vi "Configure Acquisition.vi"(8 "error in":errorcluster, 11 "Scope PXI CFG in":refnum<class "Scope PXI CFG.lvclass">) -> (0 "error out":errorcluster, 3 "Scope PXI CFG out":refnum<class "Scope PXI CFG.lvclass">)   [LabVIEW 2023, in "Scope.lvlib" / "Scope PXI.lvlib" / "Scope PXI CFG.lvclass"]
uses:
  Scope PXI CFG.lvclass
  <instrlib>/niScope/Controls/niScope acquisition type.ctl
  Scope PXI CFG.lvclass/Scope PXI CFG.ctl
  Configuration Base/Configuration Base.lvclass/Configuration Base.ctl
  33e6a676-ff2b-4197-9c74-0448942d65be.vi
  <vilib>/JDP Science/JSONtext/Next JSON Value.vi
  <vilib>/JDP Science/JSONtext/String Subset.vi
  <vilib>/JDP Science/JSONtext/Parsing/Advance past next JSON Value (inlined COPY).vi
  <vilib>/JDP Science/JSONtext/Parsing/Advance past whitespace.vi
  <vilib>/JDP Science/JSONtext/Parsing/Advance past String.vi
  <vilib>/JDP Science/JSONtext/Parsing/Advance past Number.vi
  <vilib>/JDP Science/JSONtext/Parsing/Advance past Line Ending.vi
  <vilib>/JDP Science/JSONtext/Parsing/Parse Full Path or Item Name.vi
  <vilib>/JDP Science/JSONtext/Parsing/Advance past Array.vi
  <vilib>/JDP Science/JSONtext/Parsing/Advance past Object.vi
  <vilib>/JDP Science/JSONtext/support/Error Cluster From Code.vi
  <vilib>/JDP Science/JSONtext/Offset/Find Item Locations by Path.vi
  <vilib>/JDP Science/JSONtext/JSON text to Variant.vi
  <vilib>/Utility/error.llb/Error Cluster From Error Code.vi
  <vilib>/JDP Science/JSONtext/LVClass Serializer/JSONtext LVClass Serializer.lvclass
  <vilib>/ErrorRing/Error Ring.xnode
  Configuration Base/Configuration Base.lvclass
  <vilib>/JDP Science/JSONtext/JSONtext.lvlib
panel:
  out "acquisition Type":T1 caption="acquisition type (Normal)" items=["Normal"=0, "Flex Res"=1, "DDC"=3]
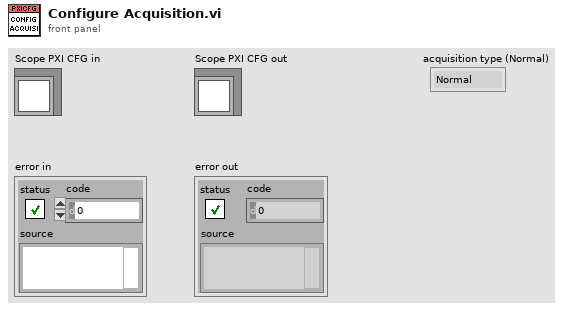
[diagram p1: front panel]
types:
  T1 = typedef "niScope acquisition type.ctl" = i32
  T2 = typedef "LVStringsAndValuesArrayTypeDef_I32.ctl" = cluster{"String":string, "Value":i32}[]
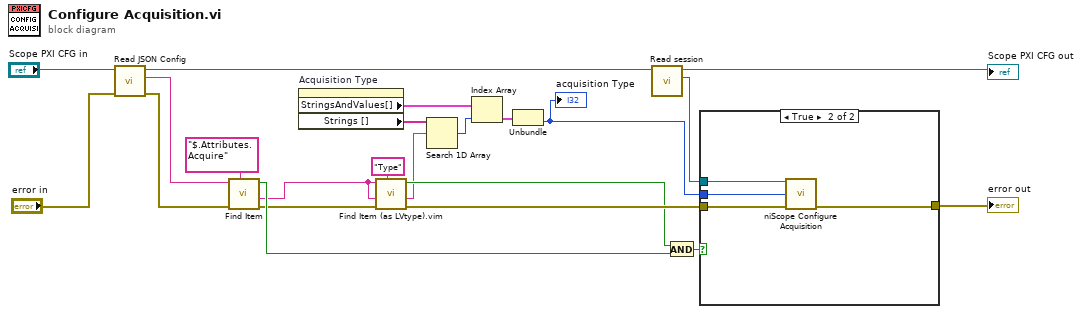
[diagram p0: block diagram]
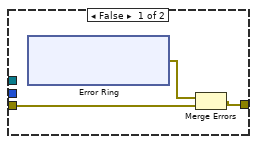
[diagram p2: hidden frame]
diagram:
  n1 = call "Read JSON Config.vi"("error in"="error in", "object in"="Scope PXI CFG in") -> ("error out"=w20:errorcluster, "<JSON>Config"=w21:string, "object out"=w22:refnum<class "Scope PXI CFG.lvclass">)  [unwired: 7 in]
  n2 = call <vilib>:"Find Item.vi"("$Path or Item Name"="$.Attributes.Acquire", "error in (no error)"=w20, "JSON"=w21) -> ("error out"=w17:errorcluster, "<JSON>"=w1:string, "Found"=w19:bool)  [unwired: 5 in, 1 out]
  n3 = property on="Acquisition Type" class="Ring (strict)"() -> ("StringsAndValues[]"=w5:T2, "Strings []"=w7:string[])  [unwired: 2 in, 2 out]
  n4 = call "Find Item (as LVtype).vim"("$Path or Item Name"="Type", "error in (no error)"=w17, "Data Type and Default Value"=w1, "JSON"=w1) -> ("error out"=w14:errorcluster, "Data"=w6:string, "Found"=w13:bool)  [unwired: 4 in, 1 out]
  n5 = Search 1D Array(1D array=w7, element=w6) -> (index of element=w4:i32)  [unwired: 1 in]
  n6 = Index Array(array=w5, index=w4) -> (element=w3:cluster{"String":string, "Value":i32})
  n7 = Unbundle(w3) -> ("Value"=w2:i32)  [unwired: 1 out]
  "acquisition Type" <- w2
  n8 = call "Read session.vi"("Scope PXI CFG in"=w22) -> ("session"=w16:refnum<k15>, "Scope PXI CFG out"=→"Scope PXI CFG out":refnum<class "Scope PXI CFG.lvclass">)  [unwired: 8 in, 1 out]
  n9 = And(x=w13, y=w19) -> (x .and. y?=w12:bool)
  n10 = case shown="True" w12 {
    tunnel: w16 -> [_ w32]
    tunnel: w14 -> [w24 w34]
    tunnel: w2 -> [_ w31]
    tunnel: [w23 w33] -> w9
    frame False {
      n11 = xnode "Error Ring"() -> ("error out"=w25:errorcluster)
      n12 = Merge Errors(w25, w24) -> (w23:errorcluster)
    }
    frame True {
      n13 = call <instrlib>:"niScope Configure Acquisition.vi"("instrument handle"=w32, "acquisition Type"=w31, "error in"=w34) -> ("error out"=w33:errorcluster)  [unwired: 11 in, 1 out]
    }
  }
  "error out" <- w9
